vi "Read Configuration Data.vi"(8 "error in (no error)":errorcluster, 11 "Path":path) -> (0 "error out":errorcluster, 2 "Configuration Settings":T1={"Offset"=0.0, "Signal Type"=enum."Sine Wave", "Frequency"=10.0, "Amplitude"=1.0, "Phase"=0.0, "Noise Amplitude"=1.0} {"Noise Amplitude" format="%.2p"; "Phase" format="%.2p"; "Amplitude" format="%0.2p"; "Frequency" format="%0.2p"; "Offset" format="%0.2p"})   [LabVIEW 2020]
uses:
  Controls/Configuration Settings.ctl
  <vilib>/Utility/config.llb/Read Key (Double).vi
  <vilib>/Utility/config.llb/Read Key (U32).vi
  <vilib>/Utility/config.llb/NI_LVConfig.lvlib
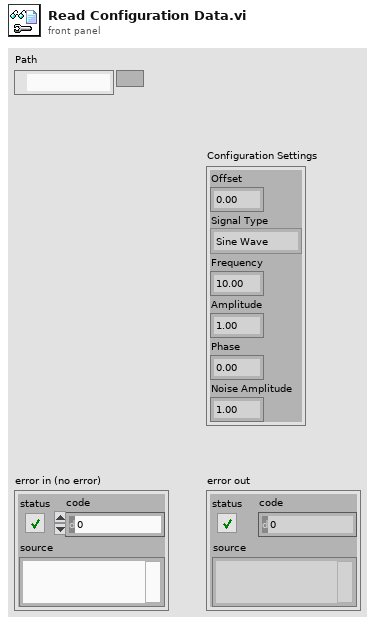
[diagram p1: front panel]
types:
  T1 = typedef "Configuration Settings.ctl" = cluster{"Offset":dbl, "Signal Type":enum16{"Sine Wave", "Triangle Wave", "Square Wave", "Sawtooth Wave"}, "Frequency":dbl, "Amplitude":dbl, "Phase":dbl, "Noise Amplitude":dbl}
  T2 = enum16{"Sine Wave", "Triangle Wave", "Square Wave", "Sawtooth Wave"}
  T3 = typedef "NI_LVConfig.lvlib/Config Data RefNum.ctl" = refnum<k1>
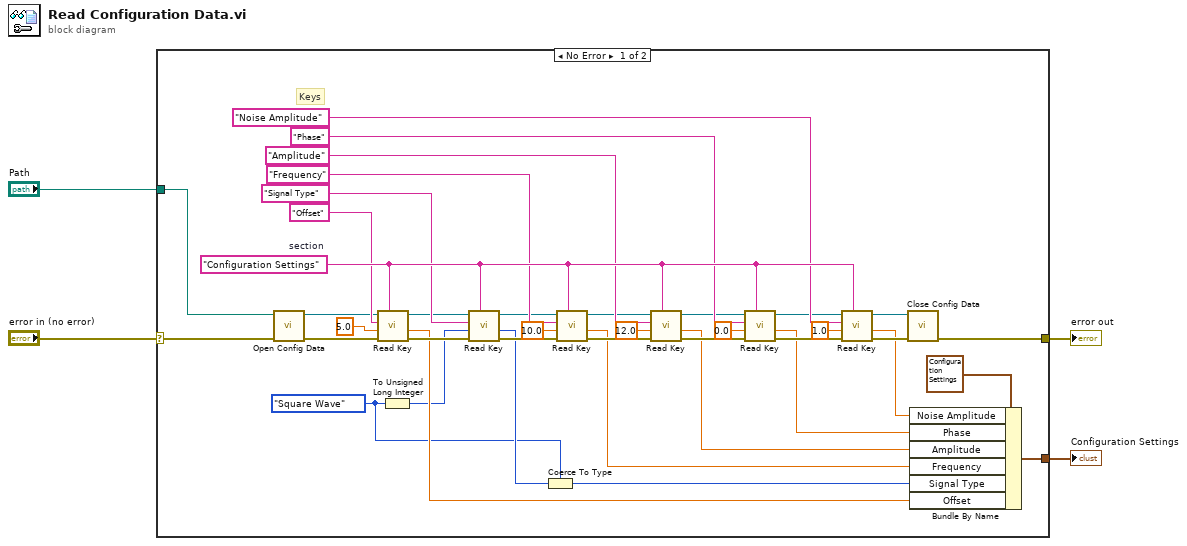
[diagram p0: block diagram]
diagram:
  n1 = case shown="No Error" "error in (no error)" {
    selector: "error in (no error)" -> [w43 w45]
    tunnel: [w42 w45] -> w3
    tunnel: "Path" -> [w44 _]
    tunnel: [w40 _] -> w1
    frame No Error {
      w5 = T2."Square Wave" ("Signal Type")
      w39 = "Configuration Settings"  # section
      # "Keys"
      n2 = call <vilib>:"Open Config Data.vi"("error in (no error)"=w43, "configuration file path"=w44) -> ("error out"=w29:errorcluster, "refnum"=w32:T3)  [unwired: 7 in, 1 out]
      n3 = call-poly <vilib>:"Read Key.vi"("section"=w39, "error in (no error)"=w29, "default value"=5.0, "key"="Offset" ("Key"), "refnum"=w32) -> ("error out"=w28:errorcluster, "value"=w18:dbl, "refnum out"=w31:T3)  [unwired: 3 in, 1 out]
      n4 = To Unsigned Long Integer(number=w5) -> (unsigned 32bit integer=w7:u32)
      n5 = call-poly <vilib>:"Read Key.vi"("section"=w39, "error in (no error)"=w28, "default value"=w7, "key"="Signal Type" ("Key"), "refnum"=w31) -> ("error out"=w27:errorcluster, "value"=w17:u32, "refnum out"=w30:T3)  [unwired: 3 in, 1 out]
      n6 = Coerce To Type(0:w17, 1:w5) -> (2:w6:T2)
      n7 = call-poly <vilib>:"Read Key.vi"("section"=w39, "error in (no error)"=w27, "default value"=10.0, "key"="Frequency" ("Key"), "refnum"=w30) -> ("error out"=w25:errorcluster, "value"=w16:dbl, "refnum out"=w26:T3)  [unwired: 3 in, 1 out]
      n8 = call-poly <vilib>:"Read Key.vi"("section"=w39, "error in (no error)"=w25, "default value"=12.0, "key"="Amplitude" ("Key"), "refnum"=w26) -> ("error out"=w23:errorcluster, "value"=w15:dbl, "refnum out"=w24:T3)  [unwired: 3 in, 1 out]
      n9 = call-poly <vilib>:"Read Key.vi"("section"=w39, "error in (no error)"=w23, "default value"=0.0, "key"="Phase" ("Key"), "refnum"=w24) -> ("error out"=w21:errorcluster, "value"=w14:dbl, "refnum out"=w22:T3)  [unwired: 3 in, 1 out]
      n10 = call-poly <vilib>:"Read Key.vi"("section"=w39, "error in (no error)"=w21, "default value"=1.0, "key"="Noise Amplitude" ("Key"), "refnum"=w22) -> ("error out"=w19:errorcluster, "value"=w13:dbl, "refnum out"=w20:T3)  [unwired: 3 in, 1 out]
      n11 = call <vilib>:"Close Config Data.vi"("error in (no error)"=w19, "refnum"=w20) -> ("error out"=w42:errorcluster)  [unwired: 8 in, 1 out]
      n12 = Bundle By Name(cluster=T1 {"Offset"=0.0, "Signal Type"=enum."Sine Wave", "Frequency"=10.0, "Amplitude"=1.0, "Phase"=0.0, "Noise Amplitude"=1.0} ("Configuration Settings"), "Noise Amplitude"=w13, "Phase"=w14, "Amplitude"=w15, "Frequency"=w16, "Signal Type"=w6, "Offset"=w18) -> (w40:T1)
    }
    frame Error {
    }
  }
  "error out" <- w3
  "Configuration Settings" <- w1
